vi "Set121dbAtten.vi"(8 "error in (no error)":errorcluster, 11 "Attenuation (dB)":i32=121 min=0 max=121 step=1) -> (0 "error out":errorcluster, 2 "Verfied":bool, 3 "Active Attenuators":bool[](array[boolean])=[FALSE, TRUE, TRUE, TRUE, TRUE, TRUE, TRUE, TRUE, TRUE])   [LabVIEW 2012]
doc: "Parses the requested attenuation then builds the SCPI command list"
panel:
  out "Open Switches - Active Attenuators":string="7161,7162,7163,7164,7165,7166,7167,7168"
  out "Closed Switches - inactive attenuators":string
  # "121 dB Attenuator Switch"
  # "1 dB"
  # "2 dB"
  # "4 dB"
  # "4 dB"
  # "10 dB"
  # "20 dB"
  # "40 dB"
  # "40 dB"
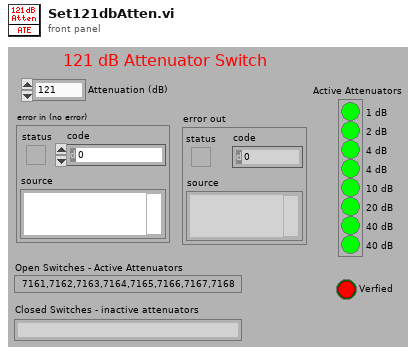
[diagram p1: front panel]
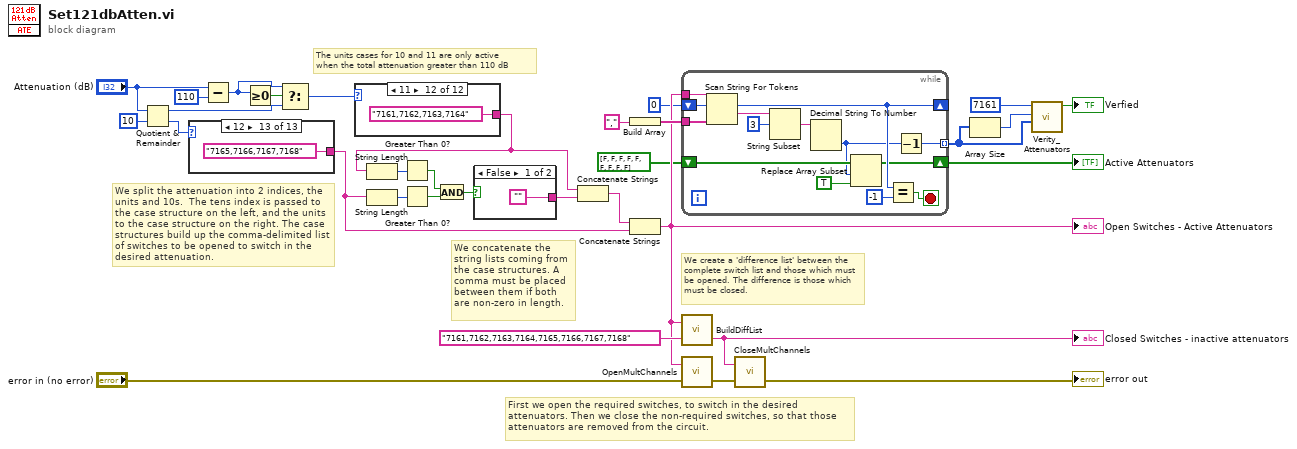
[diagram p0: block diagram]
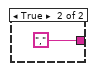
[diagram p2: hidden frame]
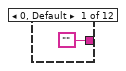
[diagram p3: hidden frame]
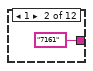
[diagram p4: hidden frame]
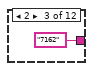
[diagram p5: hidden frame]
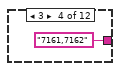
[diagram p6: hidden frame]
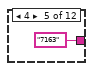
[diagram p7: hidden frame]
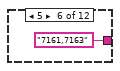
[diagram p8: hidden frame]
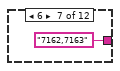
[diagram p9: hidden frame]
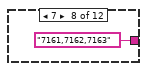
[diagram p10: hidden frame]
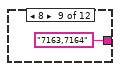
[diagram p11: hidden frame]
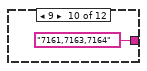
[diagram p12: hidden frame]
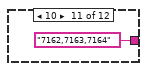
[diagram p13: hidden frame]
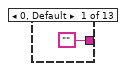
[diagram p14: hidden frame]
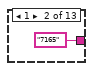
[diagram p15: hidden frame]
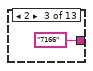
[diagram p16: hidden frame]
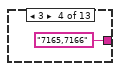
[diagram p17: hidden frame]
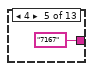
[diagram p18: hidden frame]
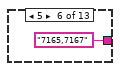
[diagram p19: hidden frame]
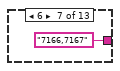
[diagram p20: hidden frame]
diagram:
  # "The units cases for 10 and 11 are only active\nwhen the total attenuation greater than 110 dB"
  # "First we open the required switches, to switch in the desired attenuators. Then we close the non-required switches, so that those attenuators are removed from the circuit."
  # "We create a 'difference list' between the complete switch list and those which must be opened. The difference is those which must be closed."
  # "We concatenate the string lists coming from the case structures. A comma must be placed between them if both are non-zero in length."
  # "We split the attenuation into 2 indices, the units and 10s.  The tens index is passed to the case structure on the left, and the units to the case structure on the right. The case structures build up the comma-delimited list of switches to be opened to switch in the desired attenuation."
  n1 = Quotient & Remainder(x="Attenuation (dB)", y=10) -> (x-y*floor(x/y)=w17:i32, floor(x/y)=w18:i32)
  n2 = case shown="12" w18 {
    tunnel: ["" "7165" "7166" "7165,7166" "7167" "7165,7167" "7166,7167" "7165,7166,7167" "7167,7168" "7165,7167,7168" "7166,7167,7168" "7165,7166,7167,7168" "7165,7166,7167,7168"] -> w11
    frame 0, Default {
    }
    frame 1 {
    }
    frame 2 {
    }
    frame 3 {
    }
    frame 4 {
    }
    frame 5 {
    }
    frame 6 {
    }
    frame 7 {
    }
    frame 8 {
    }
    frame 9 {
    }
    frame 10 {
    }
    frame 11 {
    }
    frame 12 {
    }
  }
  n3 = Subtract(x="Attenuation (dB)", y=110) -> (x-y=w13:i32)
  n4 = Greater Or Equal To 0?(x=w13) -> (x >= 0?=w14:bool)
  n5 = Select(t=w13, s=w14, f=w17) -> (s? t:f=w12:i32)
  n6 = case shown="11" w12 {
    tunnel: ["" "7161" "7162" "7161,7162" "7163" "7161,7163" "7162,7163" "7161,7162,7163" "7163,7164" "7161,7163,7164" "7162,7163,7164" "7161,7162,7163,7164"] -> w28
    frame 0, Default {
    }
    frame 1 {
    }
    frame 2 {
    }
    frame 3 {
    }
    frame 4 {
    }
    frame 5 {
    }
    frame 6 {
    }
    frame 7 {
    }
    frame 8 {
    }
    frame 9 {
    }
    frame 10 {
    }
    frame 11 {
    }
  }
  n7 = String Length(string=w28) -> (length=w29:i32)
  n8 = String Length(string=w11) -> (length=w32:i32)
  n9 = Greater Than 0?(x=w29) -> (x > 0?=w25:bool)
  n10 = Greater Than 0?(x=w32) -> (x > 0?=w24:bool)
  n11 = And(x=w25, y=w24) -> (x .and. y?=w27:bool)
  n12 = case shown="False" w27 {
    tunnel: ["" ","] -> w31
    frame False {
    }
    frame True {
    }
  }
  n13 = Concatenate Strings(w28, w31) -> (w30:string)
  n14 = Build Array(",") -> (w9:string[])
  n15 = Concatenate Strings(w30, w11) -> (w8:string)
  "Open Switches - Active Attenuators" <- w8
  n16 = while {
    tunnel: w9 -> [w71]
    shift-right: [w69] -> _
    shift-left: 0 ("offset") -> [w70]
    tunnel: w8 -> [w73]
    shift-right: [w62] -> w5
    shift-left: bool[] [FALSE, FALSE, FALSE, FALSE, FALSE, FALSE, FALSE, FALSE, FALSE] -> [w65]
    tunnel: [w60] -> w1 mode=indexing
    stop <- w63 stop-if-true
    n17 = Scan String For Tokens(6:w71, 8:w70, 9:w73) -> (1:w68:string, 2:w69:i32)  [unwired: 3 in, 2 out]
    n18 = String Subset(string=w68, offset (0)=3) -> (substring=w66:string)  [unwired: 1 in]
    n19 = Decimal String To Number(string=w66) -> (number=w61:i32)  [unwired: 2 in, 1 out]
    n20 = Replace Array Subset(array=w65, new element=TRUE ("new element/subarray"), index=w61) -> (w62:bool[])
    n21 = Equal?(x=w69, y=-1) -> (x = y?=w63:bool)
    n22 = Decrement(x=w61) -> (x-1=w60:i32)
  }
  "Active Attenuators" <- w5
  n23 = call "BuildDiffList.vi"("Reference list"="7161,7162,7163,7164,7165,7166,7167,7168", "Input list"=w8) -> ("Difference list"=w20:string)  [unwired: 1 in]
  "Closed Switches - inactive attenuators" <- w20
  n24 = call "OpenMultChannels.vi"("error in (no error)"="error in (no error)", "Channels to be opened"=w8) -> ("error out"=w22:errorcluster)  [unwired: 1 in]
  n25 = call "CloseMultChannels.vi"("error in (no error)"=w22, "Channels to be closed"=w20) -> ("error out"=→"error out":errorcluster)  [unwired: 1 in]
  n26 = Array Size(array=w1) -> (size(s)=w4:i32)
  n27 = call "Verity_Attenuators.vi"("Switches"=w1, "nSwitches"=w4, "Base Switch ID"=7161) -> ("Verfied"=→"Verfied":bool)  [unwired: 8 in]
